vi "Read.vi"(8 "error in (no error)":errorcluster, 11 "Mettler Settings in":T1) -> (0 "error out":errorcluster, 1 "Connection Error":bool, 2 "mass (g)":dbl, 3 "Mettler Settings out":T1)   [LabVIEW 2018, in "Mettler Toledo.lvlib"]
uses:
  Mettler Toledo.lvlib
  Controls/Settings Cluster.ctl
  <vilib>/regexp/Match Regular Expression.xnode
  <vilib>/ptbypt/NI_PtbyPt.lvlib
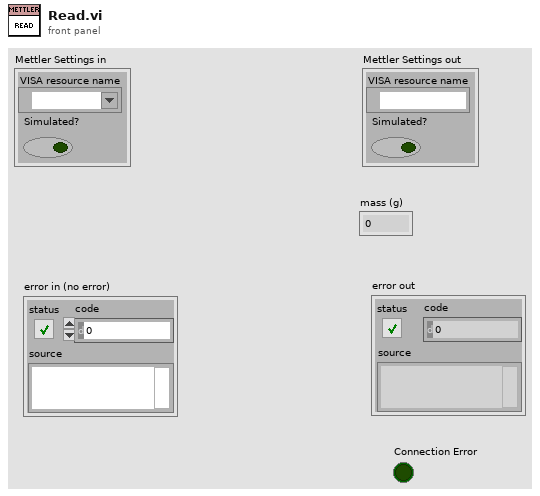
[diagram p1: front panel]
types:
  T1 = typedef "Mettler Toledo.lvlib/Settings Cluster.ctl" = cluster{"VISA resource name":refnum<visa-resource-name>, "Simulated?":bool}
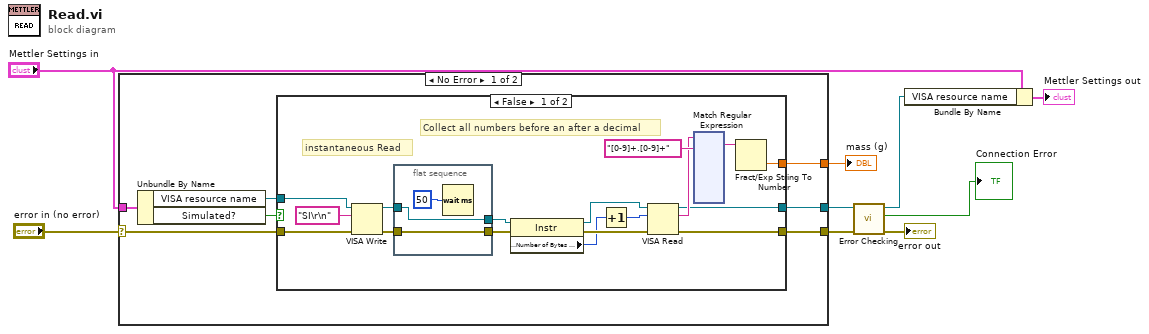
[diagram p0: block diagram]
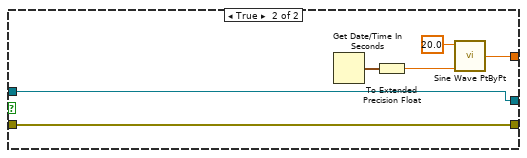
[diagram p2: hidden frame]
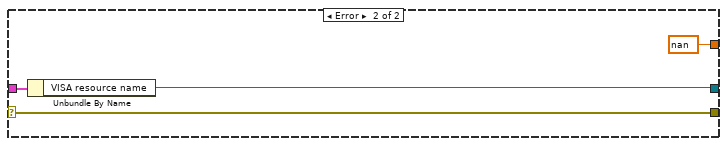
[diagram p3: hidden frame]
diagram:
  n1 = case shown="No Error" "error in (no error)" {
    selector: "error in (no error)" -> [w15 w165]
    tunnel: [w14 w165] -> w4
    tunnel: "Mettler Settings in" -> [w12 w163]
    tunnel: [w13 nan ("sine wave")] -> w7
    tunnel: [w10 w162] -> w5
    frame No Error {
      n2 = Unbundle By Name(w12) -> ("VISA resource name"=w11:refnum<visa-resource-name>, "Simulated?"=w16:bool)
      n3 = case shown="False" w16 {
        tunnel: [w19 w161] -> w14
        tunnel: w15 -> [w21 w161]
        tunnel: [w23 w157] -> w13
        tunnel: [w20 w156] -> w10
        tunnel: w11 -> [w22 w156]
        frame False {
          # "Collect all numbers before an after a decimal"
          # "instantaneous Read"
          n4 = VISA Write(VISA resource name=w22, write buffer="SI\r\n" ("Command"), error in (no error)=w21) -> (VISA resource name out=w30:refnum<visa-resource-name>, error out=w28:errorcluster)  [unwired: 1 out]
          n5 = flat-sequence {
            tunnel: [w155] -> w29
            tunnel: w30 -> [w155]
            tunnel: [w154] -> w27
            tunnel: w28 -> [w154]
            frame #0 {
              n6 = Wait (ms)(milliseconds to wait=u32 50) -> ()  [unwired: 1 out]
            }
          }
          n7 = property class="Instr"(reference=w29, error in=w27) -> (reference out=w32:refnum<visa-resource-name>, error out=w31:errorcluster, "Serial Settings:Number of Bytes at Serial Port"=w18:u32)
          n8 = Increment(x=w18) -> (x+1=w17:u32)
          n9 = VISA Read(VISA resource name=w32, byte count=w17, error in (no error)=w31) -> (VISA resource name out=w20:refnum<visa-resource-name>, read buffer=w25:string, error out=w19:errorcluster)  [unwired: 1 out]
          n10 = xnode "Match Regular Expression"("input string"=w25, "regular expression"="[0-9]+.[0-9]+" ("Regular Expression for Extracting Weight")) -> ("whole match"=w24:string)  [unwired: 4 in, 8 out]
          n11 = Fract/Exp String To Number(string=w24) -> (number=w23:dbl)  [unwired: 3 in, 1 out]
        }
        frame True {
          n12 = Get Date/Time In Seconds() -> (seconds since 1Jan1904=w160:timestamp)
          n13 = To Extended Precision Float(1:w160) -> (0:w159:ext)
          n14 = call <vilib>:"Sine Wave PtByPt.vi"("time"=w159, "amplitude"=20.0) -> ("sine wave"=w157:dbl)  [unwired: 2 in]
        }
      }
    }
    frame Error {
      n15 = Unbundle By Name(w163) -> ("VISA resource name"=w162:refnum<visa-resource-name>)
    }
  }
  "mass (g)" <- w7
  n16 = call "Error Checking.vi"("error in (no error)"=w4, "VISA resource name"=w5) -> ("error out"=→"error out":errorcluster, "Connection Error"=→"Connection Error":bool, "VISA resource name"=w2:refnum<visa-resource-name>)  [unwired: 7 in]
  n17 = Bundle By Name(cluster="Mettler Settings in", "VISA resource name"=w2) -> (→"Mettler Settings out":T1)
